vi "Parse Parameters File.vi"(8 "error in":errorcluster, 11 "path to XML document":path caption="path to parameters xml") -> (0 "error out":errorcluster, 1 "ports":T1[](array[typedef]), 3 "path to XML document out":path caption="path to parameters xml")   [LabVIEW 2020, in "ARINC 429 Import.lvlib"]
uses:
  ARINC 429 Import.lvlib
  Shared/VS Channels Definition for All Labels on Hardware Channel.ctl
  Shared/VS Channels Definition for Label.ctl
  Shared/VS Channel Definition for Parameter.ctl
  Shared/Direction.ctl
  Shared/Parameter Definition.ctl
  Encoding and Decoding/Encoding.ctl
  Shared/Transfer Type.ctl
  <vilib>/xml/Load XML File.vi
  Read Tag Element (U16).vi
  Read Tag Element (Direction).vi
  <vilib>/xml/NI_XML.lvlib
  <resource>/objmgr/DOMUserDefRef.rc
  Encoding and Decoding/Encoding and Decoding.lvlib
panel:
  out "parse errors":string
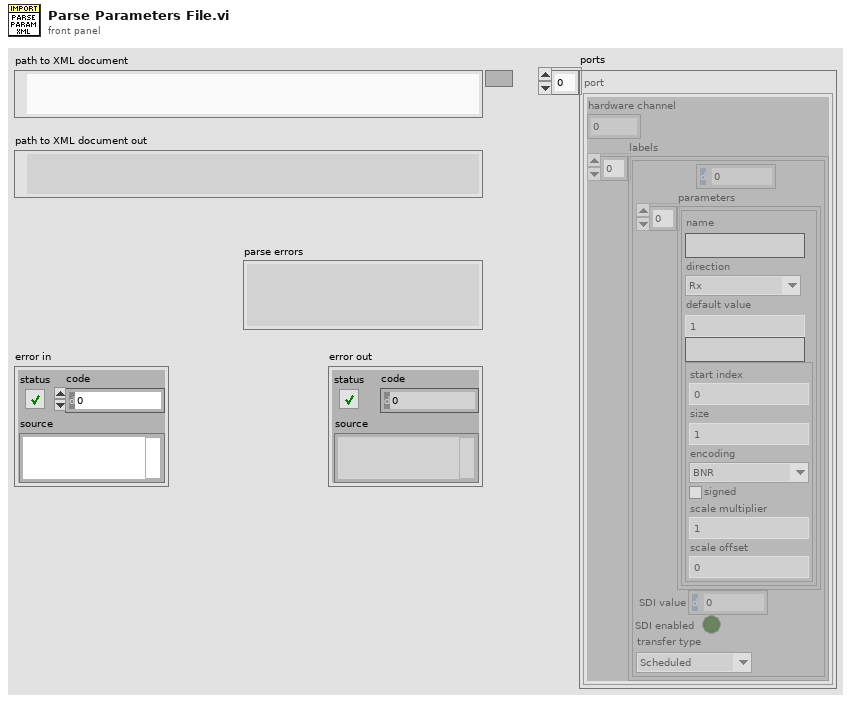
[diagram p1: front panel]
types:
  T1 = typedef "VS Channels Definition for All Labels on Hardware Channel.ctl" = cluster{"hardware channel":i32, "labels":T2[]}
  T2 = typedef "VS Channels Definition for Label.ctl" = cluster{"label (Dec)":u32, "parameters":T3[], "SDI value":u8, "SDI enabled":bool, "transfer type":T7}
  T3 = typedef "VS Channel Definition for Parameter.ctl" = cluster{"name":string, "direction":T4, "default value":dbl, "unit":string, "Parameter":T5}
  T4 = typedef "Direction.ctl" = enum16{"Rx", "Tx"}
  T5 = typedef "Parameter Definition.ctl" = cluster{"start index":i32, "size":i32, "encoding":T6, "signed":bool, "scale multiplier":dbl, "scale offset":dbl}
  T6 = typedef "Encoding and Decoding.lvlib/Encoding.ctl" = enum16{"BNR", "BCD", "Discrete"}
  T7 = typedef "Transfer Type.ctl" = enum16{"Scheduled", "Acyclic", "Block", "Strobe"}
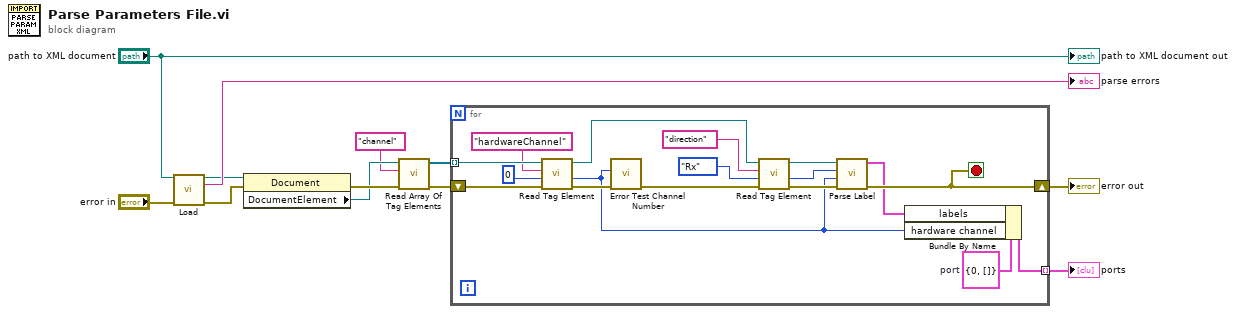
[diagram p0: block diagram]
diagram:
  n1 = call-poly <vilib>:"Load.vi"("path to XML document"="path to XML document", "error in (no error)"="error in") -> ("DOM document out"=w11:refnum<k20>, "parse errors"=→"parse errors":string, "error out"=w8:errorcluster)  [unwired: 11 in]
  n2 = property class="Document"(reference=w11, error in=w8) -> (error out=w6:errorcluster, "DocumentElement"=w5:refnum<k20>)  [unwired: 1 out]
  n3 = call "Read Array Of Tag Elements.vi"("error in"=w6, "tag name"="channel" ("Tag Name"), "node in"=w5) -> ("error out"=w7:errorcluster, "array of elements"=w4:refnum<k20>[])  [unwired: 7 in]
  n4 = for {
    tunnel: w4 -> [w29] mode=indexing
    shift-right: [w18] -> w2
    shift-left: w7 -> [w25]
    tunnel: [w28] -> w10 mode=indexing
    stop <- w18 stop-if-true
    w14 = T1 {"hardware channel"=0, "labels"=[]}  # port
    n5 = call-poly "Read Tag Element.vi"("error in"=w25, "default"=u16 0, "Tag Name"="hardwareChannel", "node in"=w29) -> ("error out"=w22:errorcluster, "value"=w13:u16, "node out"=w27:refnum<k20>)  [unwired: 5 in]
    n6 = call "Error Test Channel Number.vi"("error in"=w22, "channel #"=w13) -> ("error out"=w21:errorcluster)  [unwired: 9 in]
    n7 = call-poly "Read Tag Element.vi"("error in"=w21, "default"=Direction."Rx", "Tag Name"="direction", "node in"=w27) -> ("error out"=w20:errorcluster, "value"=w17:T4, "node out"=w19:refnum<k20>)  [unwired: 5 in]
    n8 = call "Parse Label.vi"("error in"=w20, "channel #"=w13, "direction"=w17, "node in"=w19) -> ("error out"=w18:errorcluster, "labels"=w16:T2[])  [unwired: 6 in]
    n9 = Bundle By Name(cluster=w14, "labels"=w16, "hardware channel"=w13) -> (w28:T1)
  }
  "ports" <- w10
  "error out" <- w2
  "path to XML document out" <- "path to XML document"
